vi "SmoothJitter1_10.vi"(9 "Bits in":bool[](array[boolean])=[FALSE, FALSE, FALSE, FALSE, FALSE, FALSE, FALSE, FALSE, FALSE, FALSE], 11 "Last bit in":bool) -> (1 "Smoothed bits out":bool[](array[boolean]), 3 "New last bit out":bool)   [LabVIEW 2012]
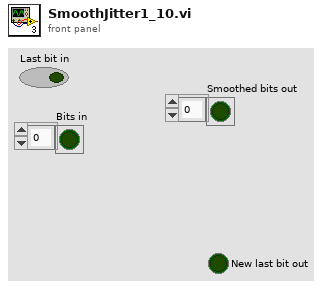
[diagram p1: front panel]
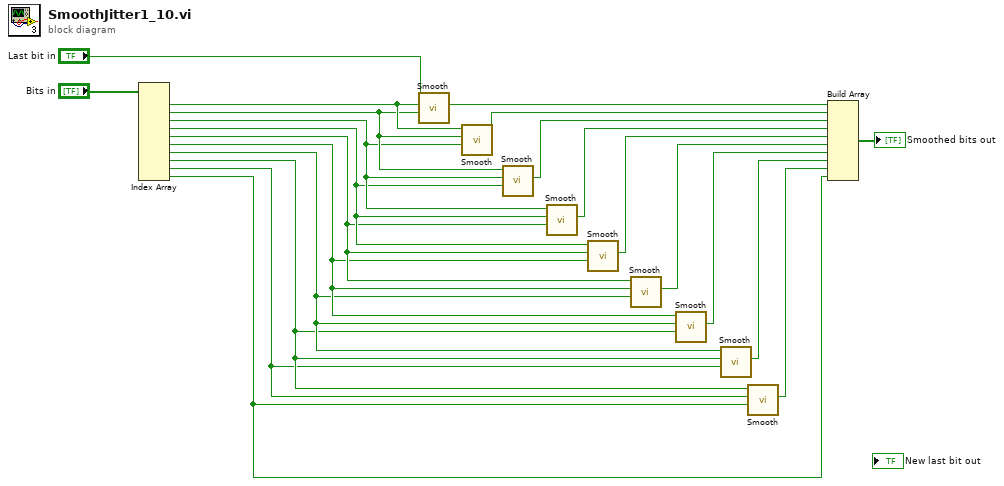
[diagram p0: block diagram]
diagram:
  n1 = Index Array(array="Bits in") -> (element #1=w18:bool, element #2=w16:bool, element #3=w14:bool, element #4=w12:bool, element #5=w10:bool, element #6=w8:bool, element #7=w6:bool, element #8=w4:bool, element #9=w3:bool, element #10=w1:bool)  [unwired: 10 in]
  n2 = call "Smooth.vi"("Bit 3"=w16, "Bit 2"=w18, "Bit 1"="Last bit in") -> ("Smooth 2"=w20:bool)  [unwired: 8 in]
  n3 = call "Smooth.vi"("Bit 3"=w14, "Bit 2"=w16, "Bit 1"=w18) -> ("Smooth 2"=w17:bool)  [unwired: 8 in]
  n4 = call "Smooth.vi"("Bit 3"=w12, "Bit 2"=w14, "Bit 1"=w16) -> ("Smooth 2"=w15:bool)  [unwired: 8 in]
  n5 = call "Smooth.vi"("Bit 3"=w10, "Bit 2"=w12, "Bit 1"=w14) -> ("Smooth 2"=w13:bool)  [unwired: 8 in]
  n6 = call "Smooth.vi"("Bit 3"=w8, "Bit 2"=w10, "Bit 1"=w12) -> ("Smooth 2"=w11:bool)  [unwired: 8 in]
  n7 = call "Smooth.vi"("Bit 3"=w6, "Bit 2"=w8, "Bit 1"=w10) -> ("Smooth 2"=w9:bool)  [unwired: 8 in]
  n8 = call "Smooth.vi"("Bit 3"=w4, "Bit 2"=w6, "Bit 1"=w8) -> ("Smooth 2"=w7:bool)  [unwired: 8 in]
  n9 = call "Smooth.vi"("Bit 3"=w3, "Bit 2"=w4, "Bit 1"=w6) -> ("Smooth 2"=w5:bool)  [unwired: 8 in]
  n10 = call "Smooth.vi"("Bit 3"=w1, "Bit 2"=w3, "Bit 1"=w4) -> ("Smooth 2"=w2:bool)  [unwired: 8 in]
  n11 = Build Array(w20, w17, w15, w13, w11, w9, w7, w5, w2, w1) -> (→"Smoothed bits out":bool[])
